vi "Delete Curve.vi"(0 "VISA resource name":refnum<visa-resource-name>, 7 "Curve to Erase (1)":i32=1 min=1 max=20 step=1, 11 "error in (no error)":errorcluster) -> (4 "VISA resource name out":refnum<visa-resource-name>, 15 "error out":errorcluster)   [LabVIEW 2019, in "Lake Shore Cryotronics 370.lvlib"]
doc: "This VI deletes the selected user curve."
uses:
  Lake Shore Cryotronics 370.lvlib
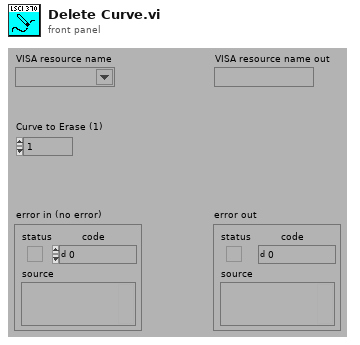
[diagram p1: front panel]
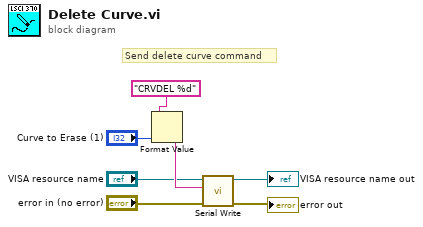
[diagram p0: block diagram]
diagram:
  # "Send delete curve command"
  n1 = Format Value(format string="CRVDEL %d", value (0)="Curve to Erase (1)") -> (output string=w3:string)  [unwired: 1 in]
  n2 = call "Serial Write.vi"("error in (no error)"="error in (no error)", "Write Buffer (\"\")"=w3, "VISA resource name"="VISA resource name") -> ("error out"=→"error out":errorcluster, "VISA resource name out"=→"VISA resource name out":refnum<visa-resource-name>)  [unwired: 6 in, 1 out]
